vi "Create Indicator.vi"(0 "Result Cluster":refnum<vi>, 5 "VI Reference":refnum<vi>, 7 "Ctl Refnum":refnum<vi>, 11 "error in (no error)":errorcluster) -> (15 "error out":errorcluster)   [LabVIEW 2021, in "Converter.lvlib"]
uses:
  Converter.lvlib
  <vilib>/Utility/miscctls.llb/LVPositionTypeDef.ctl
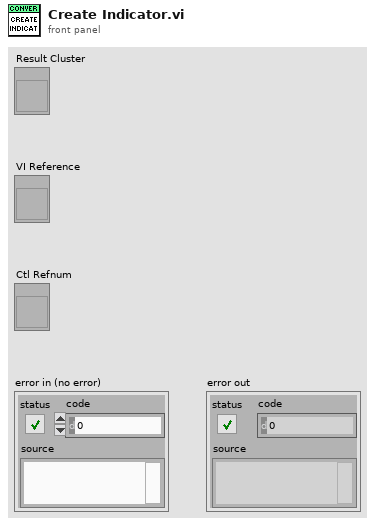
[diagram p1: front panel]
types:
  T1 = typedef "LVPositionTypeDef.ctl" = cluster{"Left":i32, "Top":i32}
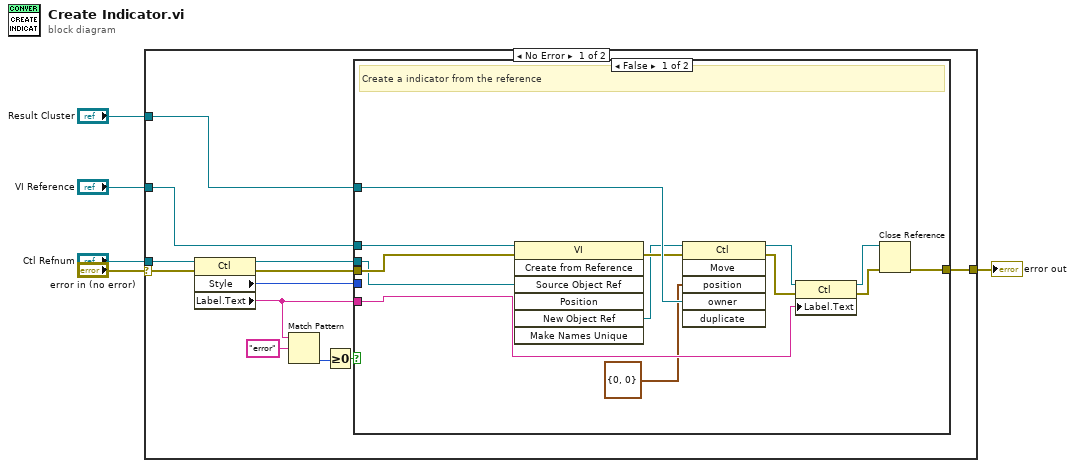
[diagram p0: block diagram]
diagram:
  n1 = case shown="No Error" "error in (no error)" {
    selector: "error in (no error)" -> [w17 w32]
    tunnel: "Ctl Refnum" -> [w16 _]
    tunnel: "VI Reference" -> [w14 _]
    tunnel: [w9 w32] -> w2
    tunnel: "Result Cluster" -> [w7 _]
    frame No Error {
      n2 = property class="Ctl"(reference=w16, error in=w17) -> (reference out=w15:refnum<vi>, error out=w8:errorcluster, "Style"=w6:u32, "Label.Text"=w10:string)
      n3 = Match Pattern(string=w10, regular expression="error") -> (offset past match=w12:i32)  [unwired: 1 in, 3 out]
      n4 = Greater Or Equal To 0?(x=w12) -> (x >= 0?=w13:bool)
      n5 = case shown="False" w13 {
        tunnel: w6 -> [_ _]
        tunnel: w7 -> [w27 _]
        tunnel: w8 -> [w30 w31]
        tunnel: w15 -> [w26 _]
        tunnel: [w29 w31] -> w9
        tunnel: w10 -> [w28 _]
        tunnel: w14 -> [w25 _]
        frame False {
          # "Create a indicator from the reference"
          n6 = invoke class="VI" method="Create from Reference"(reference=w25, error in=w30, "Source Object Ref"=w26) -> (error out=w24:errorcluster, "New Object Ref"=w23:refnum<vi>)  [unwired: 4 in, 5 out]
          n7 = invoke class="Ctl" method="Move"(reference=w23, error in=w24, "position"=T1 {"Left"=0, "Top"=0}, "owner"=w27) -> (reference out=w19:refnum<vi>, error out=w21:errorcluster)  [unwired: 2 in, 4 out]
          n8 = property class="Ctl"(reference=w19, error in=w21, "Label.Text"=w28) -> (reference out=w18:refnum<vi>, error out=w20:errorcluster)
          n9 = Close Reference(reference=w18, error in (no error)=w20) -> (error out=w29:errorcluster)
        }
        frame True {
          # "Ignore it is error indicator"
        }
      }
    }
    frame Error {
    }
  }
  "error out" <- w2
